vi "Event-Driven State Machine.vi"() -> ()   [LabVIEW 2020]
uses:
  support/State Machine Data.ctl
  support/States.ctl
  <vilib>/DAQmx/read.llb/DAQmx Read (Analog 2D DBL NChan NSamp).vi
  <vilib>/DAQmx/write.llb/DAQmx Write (Analog DBL 1Chan 1Samp).vi
  <vilib>/DAQmx/create/channels.llb/DAQmx Create Channel (AI-Voltage-Basic).vi
  <vilib>/DAQmx/configure/timing.llb/DAQmx Timing (Sample Clock).vi
  <vilib>/DAQmx/miscellaneous.llb/DAQmx Fill In Error Info.vi
  <vilib>/Utility/file.llb/Write Delimited Spreadsheet (DBL).vi
  <vilib>/DAQmx/create/channels.llb/DAQmx Create Channel (AO-Voltage-Basic).vi
panel:
  out "RMS Results Per Channel":dbl[](array[numeric])
  out "Threshold exceeded?":bool
  in  "Acquire":bool
  in  "Samples per channel":i32=100
  in  "Sample Rate":dbl=1000.0
  in  "AI Voltage Channel":tag="PCI-6221/ai0, PCI-6221/ai2:3"
  in  "AO Voltage Channel":tag="PCI-6221/ao0"
  in  "Generate Stimulus":bool
  in  "Threshold (rms)":dbl=1.0
  in  "Clear":bool
  in  "Exit":bool
  out "Graph":dbl[][](graph)
  # "Analysis"
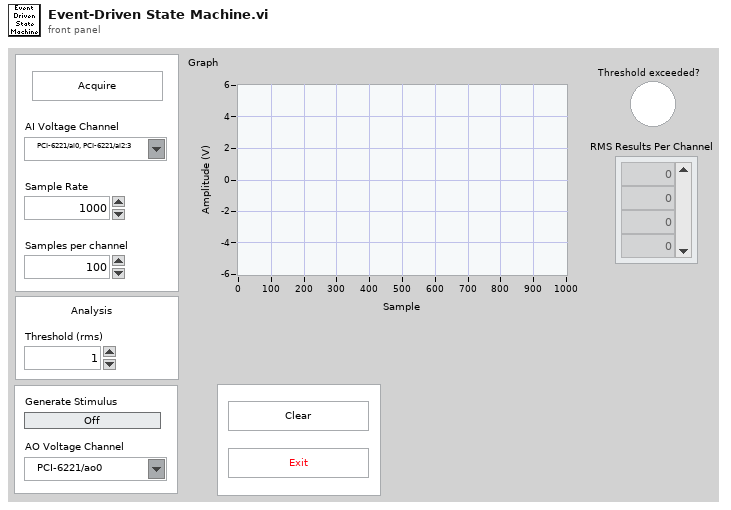
[diagram p1: front panel]
types:
  T1 = typedef "States.ctl" = enum16{"Initialize", "Wait for Event", "Acquire", "Analyze", "Log", "Clear", "Update Stimulus", "Update UI", "Exit"}
  T2 = typedef "State Machine Data.ctl" = cluster{"Acquisition Data":dbl[][], "Stimulus Value":bool}
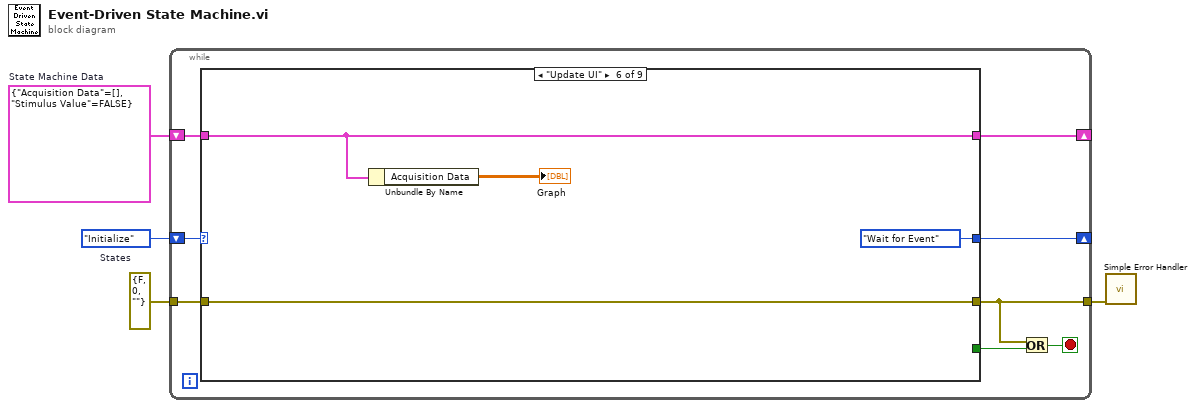
[diagram p0: block diagram]
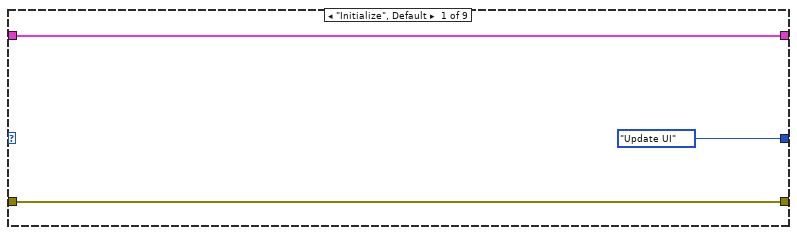
[diagram p2: hidden frame]
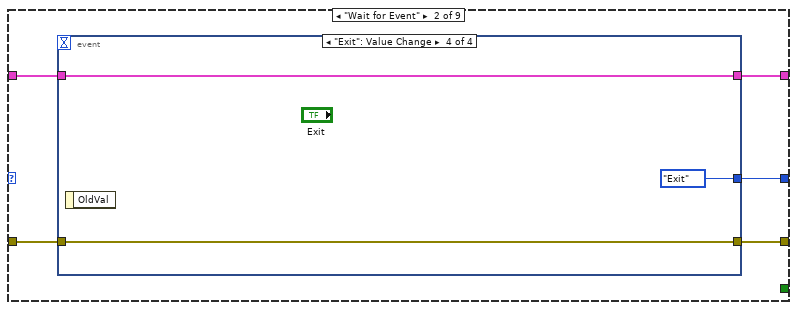
[diagram p3: hidden frame]
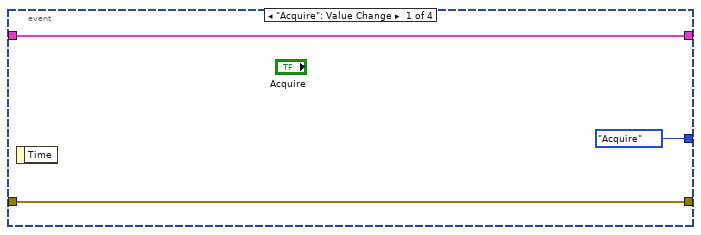
[diagram p4: hidden frame]
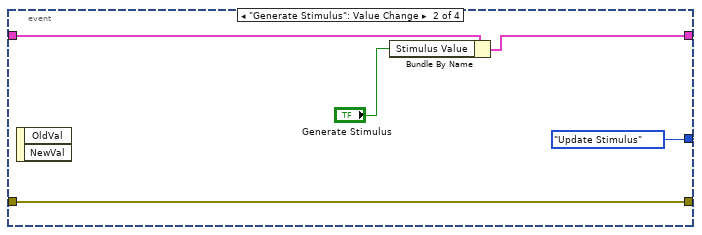
[diagram p5: hidden frame]
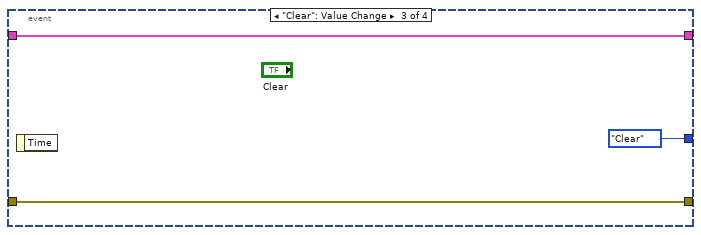
[diagram p6: hidden frame]
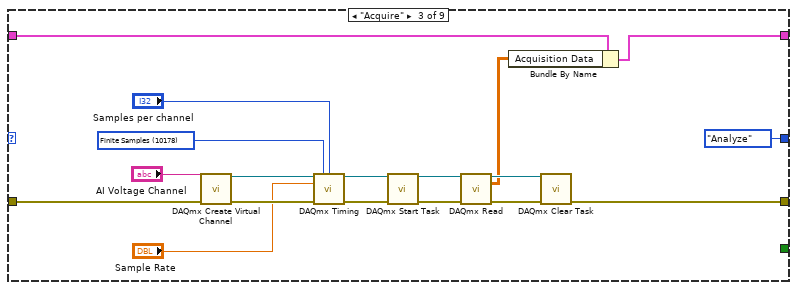
[diagram p7: hidden frame]
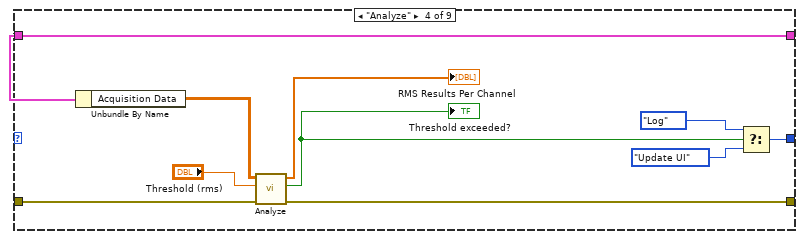
[diagram p8: hidden frame]
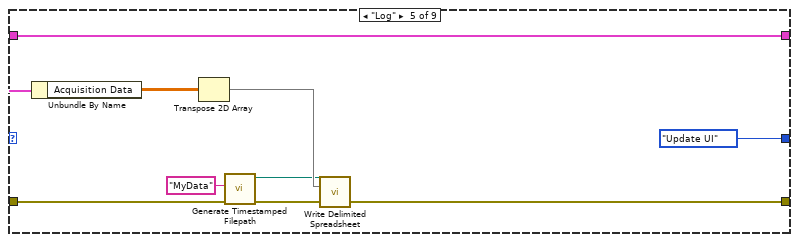
[diagram p9: hidden frame]
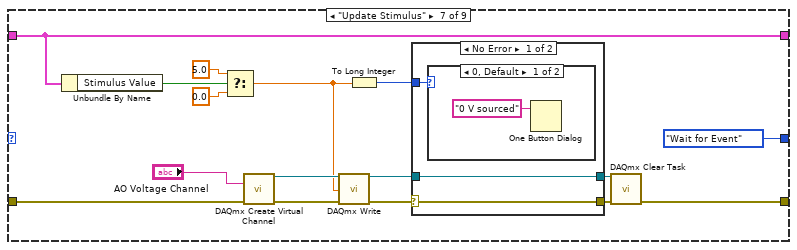
[diagram p10: hidden frame]
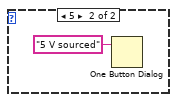
[diagram p11: hidden frame]
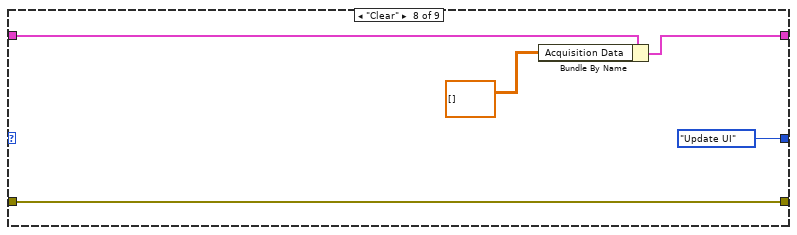
[diagram p13: hidden frame]
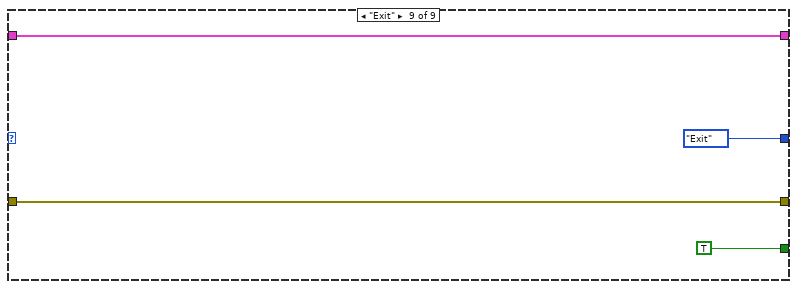
[diagram p14: hidden frame]
diagram:
  w4 = States."Initialize"  # States
  w3 = T2 {"Acquisition Data"=[], "Stimulus Value"=FALSE}  # State Machine Data
  n1 = while {
    shift-right: [w9] -> _
    shift-left: w4 -> [w12]
    shift-right: [w10] -> _
    shift-left: w3 -> [w11]
    tunnel: errorcluster {"status"=FALSE, "code"=0, "source"=""} ("error constant") -> [w8]
    tunnel: [w7] -> w1
    stop <- w5 stop-if-true
    n2 = case shown="\"Update UI\"" w12 {
      tunnel: w11 -> [w15 w20 w40 w62 w70 w74 w91 w102 w106]
      tunnel: [w15 w19 w36 w62 w70 w74 w91 w100 w106] -> w10
      tunnel: [States."Update UI" ("States") w16 States."Analyze" ("States") w54 States."Update UI" ("States") States."Wait for Event" ("States") States."Wait for Event" ("States") States."Update UI" ("States") States."Exit" ("States")] -> w9
      tunnel: w8 -> [w13 w18 w52 w59 w68 w75 w85 w103 w107]
      tunnel: [w13 w17 w38 w57 w64 w75 w86 w103 w107] -> w7
      tunnel: [_ _ _ _ _ _ _ _ TRUE] -> w6
      frame "Initialize", Default {
      }
      frame "Wait for Event" {
        n3 = event shown="[3] \"Exit\": Value Change" {
          selector: _ -> [_ _ _ _]
          dyn-events: _ -> [_ _ _ _]
          timeout: _ -> [_ _ _ _]
          tunnel: w20 -> [w22 w28 w31 w33]
          tunnel: [w22 w27 w31 w33] -> w19
          tunnel: w18 -> [w23 w26 w30 w34]
          tunnel: [w23 w26 w30 w34] -> w17
          tunnel: [States."Acquire" ("Enum") States."Update Stimulus" ("Enum") States."Clear" ("Enum") States."Exit" ("Enum")] -> w16
          event "Acquire": Value Change {
            n4 = event-data() -> ()  [unwired: 1 in, 1 out]
          }
          event "Generate Stimulus": Value Change {
            n5 = event-data() -> ()  [unwired: 1 in, 2 out]
            n6 = Bundle By Name(cluster=w28, "Stimulus Value"="Generate Stimulus") -> (w27:T2)
          }
          event "Clear": Value Change {
            n7 = event-data() -> ()  [unwired: 1 in, 1 out]
          }
          event "Exit": Value Change {
            n8 = event-data() -> ()  [unwired: 1 in, 1 out]
          }
        }
      }
      frame "Acquire" {
        w48 = 10178 items=["Finite Samples"=10178, "Continuous Samples"=10123, "Hardware Timed Single Point"=12522] ("sample mode")
        n9 = call-poly <vilib>:"DAQmx Create Virtual Channel.vi"("physical channels"="AI Voltage Channel", "error in"=w52) -> ("task out"=w49:refnum<k21>, "error out"=w50:errorcluster)  [unwired: 12 in]
        n10 = call-poly <vilib>:"DAQmx Timing.vi"("task/channels in"=w49, "sample mode"=w48, "samples per channel"="Samples per channel", "rate"="Sample Rate", "error in"=w50) -> ("task out"=w46:refnum<k21>, "error out"=w45:errorcluster)  [unwired: 9 in]
        n11 = call <vilib>:"DAQmx Start Task.vi"("task/channels in"=w46, "error in"=w45) -> ("task out"=w44:refnum<k21>, "error out"=w43:errorcluster)  [unwired: 12 in]
        n12 = call-poly <vilib>:"DAQmx Read.vi"("task/channels in"=w44, "error in"=w43) -> ("task out"=w42:refnum<k21>, "data"=w39:dbl[][], "error out"=w41:errorcluster)  [unwired: 11 in]
        n13 = Bundle By Name(cluster=w40, "Acquisition Data"=w39) -> (w36:T2)
        n14 = call <vilib>:"DAQmx Clear Task.vi"("task in"=w42, "error in"=w41) -> ("error out"=w38:errorcluster)  [unwired: 13 in]
      }
      frame "Analyze" {
        n15 = Unbundle By Name(w62) -> ("Acquisition Data"=w61:dbl[][])
        n16 = call "Analyze.vi"("error in (no error)"=w59, "Threshold (rms)"="Threshold (rms)", "N-Channel Data (2D DBL)"=w61) -> ("error out"=w57:errorcluster, "Threshold Exceeded?"=w53:bool, "N-Channel RMS Results"=→"RMS Results Per Channel":dbl[])  [unwired: 5 in, 1 out]
        "Threshold exceeded?" <- w53
        n17 = Select(t=States."Log" ("States"), s=w53, f=States."Update UI" ("States")) -> (s? t:f=w54:T1)
      }
      frame "Log" {
        n18 = Unbundle By Name(w70) -> ("Acquisition Data"=w71:dbl[][])
        n19 = Transpose 2D Array(2D array=w71) -> (transposed array=w67:dbl[][])
        n20 = call "Generate Timestamped Filepath.vi"("Error In"=w68, "appended filename"="MyData") -> ("Error Out"=w65:errorcluster, "timestamped relative filepath"=w66:path)  [unwired: 8 in]
        n21 = call-poly <vilib>:"Write Delimited Spreadsheet.vi"("file path (dialog if empty)"=w66, "2D data"=w67, "error in (no error)"=w65) -> ("error out"=w64:errorcluster)  [unwired: 11 in, 1 out]
      }
      frame "Update UI" {
        n22 = Unbundle By Name(w74) -> ("Acquisition Data"=→"Graph":dbl[][])
      }
      frame "Update Stimulus" {
        n23 = Unbundle By Name(w91) -> ("Stimulus Value"=w82:bool)
        n24 = Select(t=5.0, s=w82, f=0.0) -> (s? t:f=w81:dbl)
        n25 = call-poly <vilib>:"DAQmx Create Virtual Channel.vi"("physical channels"="AO Voltage Channel", "error in"=w85) -> ("task out"=w88:refnum<k21>, "error out"=w87:errorcluster)  [unwired: 12 in]
        n26 = call-poly <vilib>:"DAQmx Write.vi"("task/channels in"=w88, "data"=w81, "error in"=w87) -> ("task out"=w78:refnum<k21>, "error out"=w79:errorcluster)  [unwired: 10 in, 1 out]
        n27 = To Long Integer(number=w81) -> (32bit integer=w80:i32)
        n28 = case shown="No Error" w79 {
          selector: w79 -> [w92 w97]
          tunnel: w80 -> [w94 _]
          tunnel: w78 -> [w93 w98]
          tunnel: [w93 w98] -> w77
          tunnel: [w92 w97] -> w76
          frame No Error {
            n29 = case shown="0, Default" w94 {
              frame 0, Default {
                n30 = One Button Dialog(message="0 V sourced") -> ()  [unwired: 1 in, 1 out]
              }
              frame 5 {
                n31 = One Button Dialog(message="5 V sourced") -> ()  [unwired: 1 in, 1 out]
              }
            }
          }
          frame Error {
          }
        }
        n32 = call <vilib>:"DAQmx Clear Task.vi"("task in"=w77, "error in"=w76) -> ("error out"=w86:errorcluster)  [unwired: 13 in]
      }
      frame "Clear" {
        n33 = Bundle By Name(cluster=w102, "Acquisition Data"=dbl[][] []) -> (w100:T2)
      }
      frame "Exit" {
      }
    }
    n34 = Or(x=w7, y=w6) -> (x .or. y?=w5:bool)
  }
  n35 = call <vilib>:"Simple Error Handler.vi"("error in (no error)"=w1) -> ()  [unwired: 4 in, 5 out]
